vi "boolean debounce 2016.vi"(1 "Input Boolean":bool) -> (0 "Output Boolean":bool)   [LabVIEW 2016]
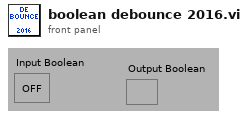
[diagram p1: front panel]
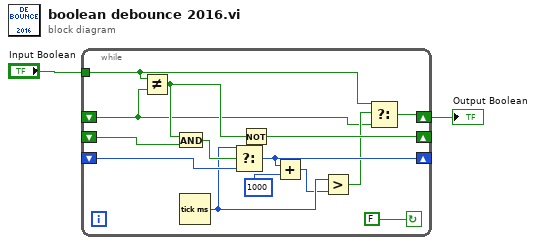
[diagram p0: block diagram]
diagram:
  n1 = while {
    shift-left: _ -> [w13]
    shift-right: [w16] -> _
    shift-left: _ -> [w15]
    shift-right: [w10] -> _
    tunnel: "Input Boolean" -> [w6]
    shift-left: _ -> [w4]
    shift-right: [w5] -> w1
    stop <- FALSE continue-if-true
    n2 = Not Equal?(x=w6, y=w4) -> (x != y?=w14:bool)
    n3 = And(x=w14, y=w13) -> (x .and. y?=w12:bool)
    n4 = Tick Count (ms)() -> (millisecond timer value=w9:u32)
    n5 = Select(t=w9, s=w12, f=w15) -> (s? t:f=w10:u32)
    n6 = Not(x=w14) -> (.not. x?=w16:bool)
    n7 = Add(x=w10, y=1000) -> (x+y=w8:u32)
    n8 = Greater?(x=w9, y=w8) -> (0:w7:bool)
    n9 = Select(t=w6, s=w7, f=w4) -> (s? t:f=w5:bool)
  }
  "Output Boolean" <- w1
